vi "SetObject.vi"(8 "ErrorIn":errorcluster, 10 "ObjectName":string, 11 "Type":refnum<class>) -> (0 "ErrorOut":errorcluster, 3 "ObjectOut":refnum<class>)   [LabVIEW 2021]
uses:
  d2c2a4a4-8417-45fa-9e2b-261bf9f1a583.vi
  <vilib>/TriekselSoft/TracerLibrary/TracerLibrary/Tracer/protected/SendMessage.vi
  <vilib>/TriekselSoft/TracerLibrary/TracerLibrary/Tracer/protected/Timestamp.vi
  d2c2a4a4-8417-45fa-9e2b-261bf9f1a583.vi/f75db090-0877-4668-94fb-75c2140b1617.vi
  <vilib>/TriekselSoft/TracerLibrary/TracerLibrary/Tracer/Tracer_Level-Debug.vi
  <vilib>/JDP Science/JSONtext/Variant to JSON Text.vi
  <vilib>/TriekselSoft/TracerLibrary/TracerLibrary/Tracer/protected/Tracer_ClassAttributes.vi
  <vilib>/JDP Science/JSONtext/LVClass Serializer/JSONtext LVClass Serializer.lvclass
  Application.lvclass
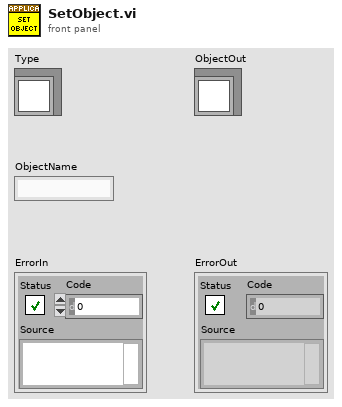
[diagram p1: front panel]
types:
  T1 = typedef "Application.lvclass/ObjectAttributes.ctl" = cluster{"Objects":variant, "BasePath":path, "Application":refnum<class "Application.lvclass">}
  T2 = cluster{"ObjectName":string, "class name":string}
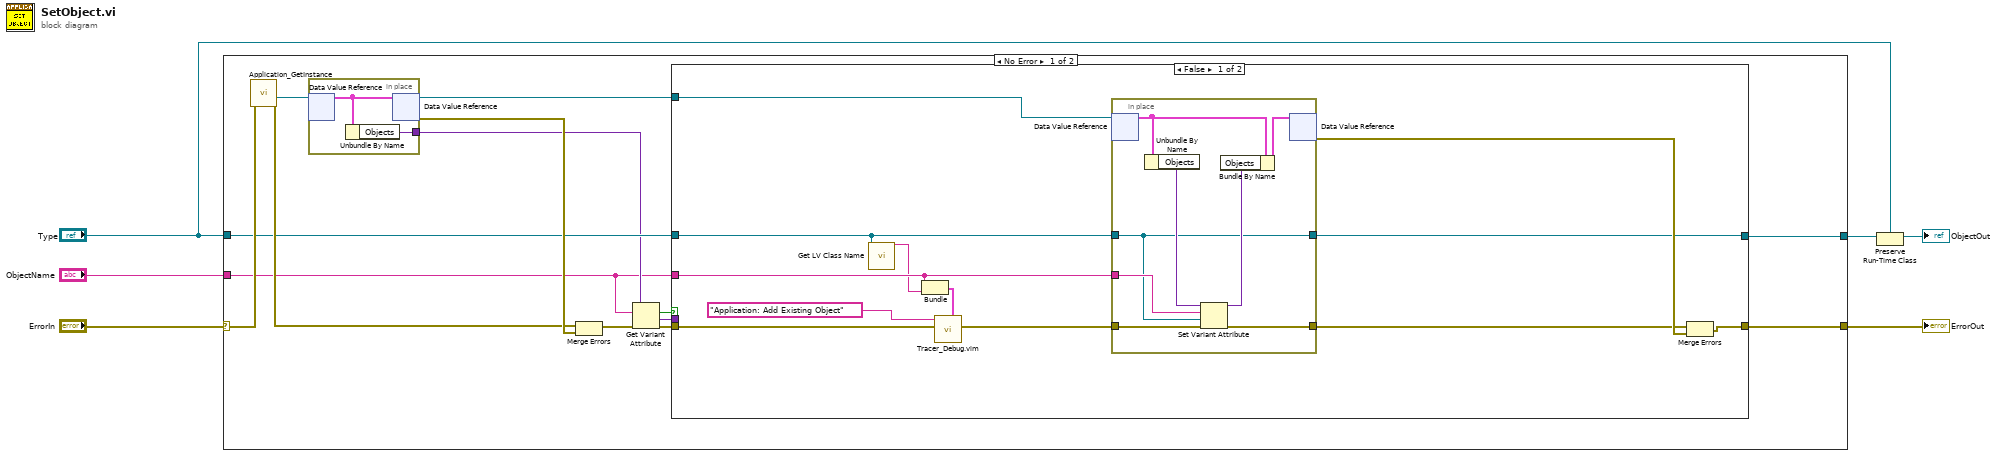
[diagram p0: block diagram]
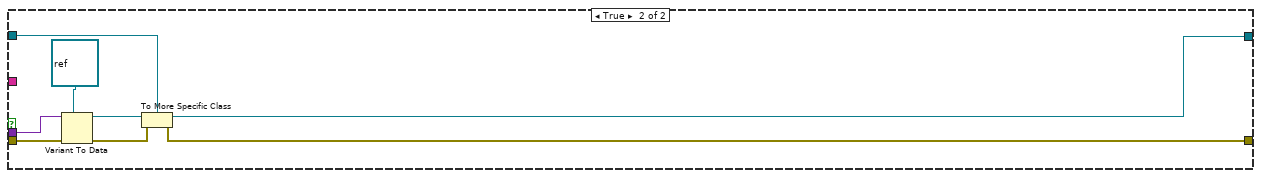
[diagram p2: hidden frame]
diagram:
  n1 = case shown="No Error" "ErrorIn" {
    selector: "ErrorIn" -> [w20 w51]
    tunnel: [w16 w51] -> w5
    tunnel: "ObjectName" -> [w7 _]
    tunnel: "Type" -> [w14 _]
    tunnel: [w13 _] -> w3
    frame No Error {
      n2 = call "Application_GetInstance.vi"("ErrorIn"=w20) -> ("ErrorOut"=w15:errorcluster, "DVRRefOut"=w12:refnum<data-value>)  [unwired: 6 in, 3 out]
      n3 = in-place {
        in-place-border: [w49] -> w9
        n4 = in-place-dvr #1(w12) -> (w50:T1)  [unwired: 1 out]
        n5 = Unbundle By Name(w50) -> ("Objects"=w49:variant)
        n6 = in-place-dvr #1(w50) -> (w8:refnum<data-value>, w19:errorcluster)
      }
      n7 = Merge Errors(w15, w19) -> (w18:errorcluster)
      n8 = Get Variant Attribute(Variant=w9, name=w7, error in=w18) -> (found=w11:bool, value=w10:variant, error out=w17:errorcluster)  [unwired: 1 in, 1 out]
      n9 = case shown="False" w11 {
        tunnel: w17 -> [w28 w48]
        tunnel: w14 -> [w24 w41]
        tunnel: [w32 w46] -> w16
        tunnel: [w26 w42] -> w13
        tunnel: w10 -> [_ w44]
        tunnel: w8 -> [w27 _]
        tunnel: w7 -> [w23 _]
        frame False {
          n10 = call <vilib>:"Get LV Class Name.vi"("object"=w24) -> ("class name"=w22:string)  [unwired: 9 in, 1 out]
          n11 = Bundle("ObjectName"=w23, "class name"=w22) -> (w21:T2)  [unwired: 1 in]
          n12 = call "Tracer_Debug.vim"("Data"=w21, "Error In"=w28, "Text"="Application: Add Existing Object" ("InfoText")) -> ("Error Out"=w29:errorcluster)  [unwired: 8 in]
          n13 = in-place {
            in-place-border: w24 -> [w33]
            in-place-border: w23 -> [w38]
            in-place-border: w29 -> [w40]
            in-place-border: [w39] -> w30
            in-place-border: [w33] -> w26
            n14 = in-place-dvr #2(w27) -> (w37:T1)  [unwired: 1 out]
            n15 = Unbundle By Name(w37) -> ("Objects"=w35:variant)
            n16 = Set Variant Attribute(Variant=w35, name=w38, value=w33, error in=w40) -> (Variant out=w34:variant, error out=w39:errorcluster)  [unwired: 1 out]
            n17 = Bundle By Name(cluster=w37, "Objects"=w34) -> (w36:T1)
            n18 = in-place-dvr #2(w36) -> (w31:errorcluster)  [unwired: 1 out]
          }
          n19 = Merge Errors(w30, w31) -> (w32:errorcluster)
        }
        frame True {
          n20 = Variant To Data(error in=w48, type=refnum<class> refnum ("Type"), Variant=w44) -> (data=w43:refnum<class>, error out=w47:errorcluster)
          n21 = To More Specific Class(target class=w41, reference=w43, error in=w47) -> (specific class reference=w42:refnum<class>, error out=w46:errorcluster)
        }
      }
    }
    frame Error {
    }
  }
  "ErrorOut" <- w5
  n22 = Preserve Run-Time Class(object in=w3, 2:"Type") -> (object out=→"ObjectOut":refnum<class>)  [unwired: 1 in, 1 out]
